vi "Generate New Data Directory.vi"(8 "error in":errorcluster, 11 "path":path=path "C:/CRD_PAS Data") -> (0 "error out":errorcluster, 3 "created path":path)   [LabVIEW 2014]
doc: "Create new directory in the a data directory. This new directory will look something like <B>yyyymmdd.x</B> where the characters represent the date folder was generated and the x represents an integer that is incremented each time a new directory is made for the day.\n\nThe directory in which all of these are stored is set to C:\\CRD_PAS_Data; if this directory does not exist, create it."
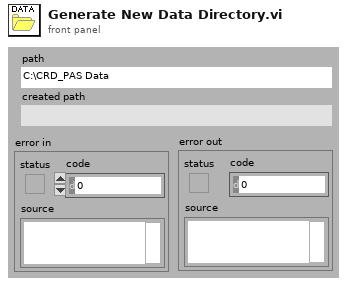
[diagram p1: front panel]
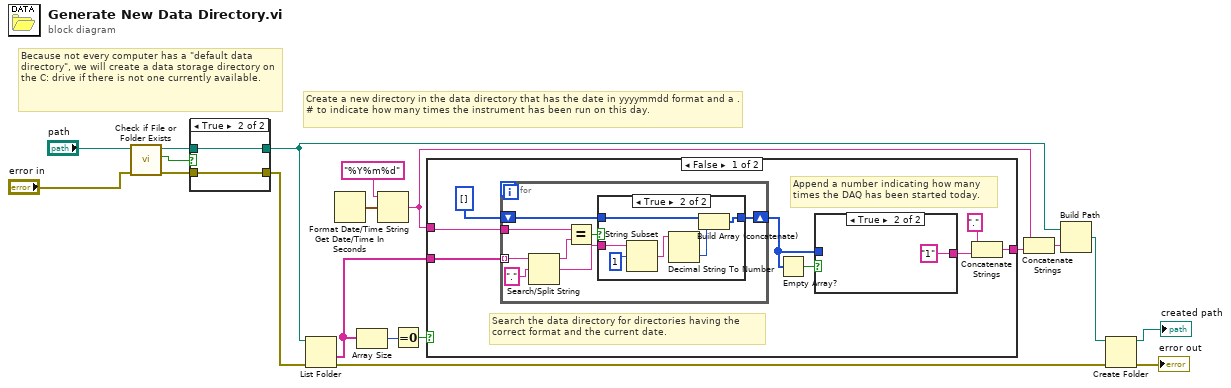
[diagram p0: block diagram]
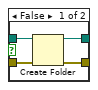
[diagram p2: hidden frame]
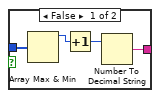
[diagram p3: hidden frame]
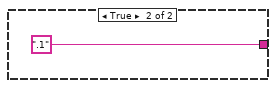
[diagram p5: hidden frame]
diagram:
  # "Create a new directory in the data directory that has the date in yyyymmdd format and a .# to indicate how many times the instrument has been run on this day."
  # "Because not every computer has a \"default data directory\", we will create a data storage directory on the C: drive if there is not one currently available."
  n1 = call <vilib>:"Check if File or Folder Exists.vi"("error in (no error)"="error in", "path"="path") -> ("error out"=w2:errorcluster, "file or folder exists?"=w6:bool, "dup path"=w4:path)  [unwired: 7 in]
  n2 = case shown="True" w6 {
    tunnel: [w22 w25] -> w5
    tunnel: w4 -> [w23 w25]
    tunnel: w2 -> [w21 w24]
    tunnel: [w20 w24] -> w1
    frame False {
      n3 = Create Folder(path (use dialog)=w23, error in=w21) -> (created path=w22:path, error out=w20:errorcluster)  [unwired: 1 in, 1 out]
    }
    frame True {
    }
  }
  n4 = List Folder(path=w5, error in=w1) -> (folder names=w15:string[], error out=w12:errorcluster)  [unwired: 4 out]
  n5 = Get Date/Time In Seconds() -> (seconds since 1Jan1904=w11:timestamp)
  n6 = Array Size(array=w15) -> (size(s)=w8:i32)
  n7 = Format Date/Time String(time format string (%c)="%Y%m%d", seconds (now)=w11) -> (date/time string=w14:string)  [unwired: 1 out]
  n8 = Equal To 0?(x=w8) -> (x = 0?=w17:bool)
  n9 = case shown="False" w17 {
    tunnel: w14 -> [w28 _]
    tunnel: w15 -> [w27 _]
    tunnel: [w26 ".1"] -> w16
    frame False {
      # "Search the data directory for directories having the correct format and the current date."
      # "Append a number indicating how many times the DAQ has been started today."
      n10 = for {
        tunnel: w27 -> [w46] mode=indexing
        shift-right: [w39] -> w29
        shift-left: i32[] [] -> [w40]
        tunnel: w28 -> [w42]
        n11 = Search/Split String(string=w46, search string/char (-)=".") -> (substring before match=w43:string, match + rest of string=w44:string)  [unwired: 2 out]
        n12 = Equal?(x=w42, y=w43) -> (x = y?=w41:bool)
        n13 = case shown="True" w41 {
          tunnel: w44 -> [_ w53]
          tunnel: w40 -> [w47 w50]
          tunnel: [w47 w49] -> w39
          frame False {
          }
          frame True {
            n14 = String Subset(string=w53, offset (0)=1) -> (substring=w51:string)  [unwired: 1 out]
            n15 = Decimal String To Number(string=w51) -> (number=w48:i32)  [unwired: 3 out]
            n16 = Build Array (concatenate)(w50, w48) -> (w49:i32[])
          }
        }
      }
      n17 = Empty Array?(array=w29) -> (empty?=w30:bool)
      n18 = case shown="True" w30 {
        tunnel: [w35 "1"] -> w33
        tunnel: w29 -> [w34 _]
        frame False {
          n19 = Array Max & Min(array=w34) -> (max value=w37:i32)  [unwired: 3 out]
          n20 = Increment(x=w37) -> (x+1=w36:i32)
          n21 = Number To Decimal String(number=w36) -> (decimal integer string=w35:string)  [unwired: 1 out]
        }
        frame True {
        }
      }
      n22 = Concatenate Strings("." ("string"), w33) -> (w26:string)
    }
    frame True {
    }
  }
  n23 = Concatenate Strings(w14, w16) -> (w9:string)
  n24 = Build Path(base path=w5, name or relative path=w9) -> (appended path=w13:path)
  n25 = Create Folder(path (use dialog)=w13, error in=w12) -> (created path=→"created path":path, error out=→"error out":errorcluster)  [unwired: 2 out]
